vi "Begin.vi"() -> (0 "No error":errorcluster)   [LabVIEW 2012]
doc: "Called before other user functions, this VI is expected to open initial I/O refnums, load in file data, and do all program initialization. Notice that the <B>error out</B> terminal is simply used for data flow. Wiring it to other structures or subVIs ensures that this VI runs first."
panel:
  out "error out":errorcluster
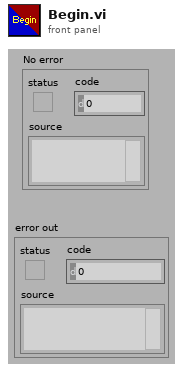
[diagram p1: front panel]
types:
  T1 = typedef "WPI_CameraDevRef.ctl" = cluster{"Camera Address":string, "CameraStatus":errorcluster, "Acquire Image Notifier":refnum<notifier>}
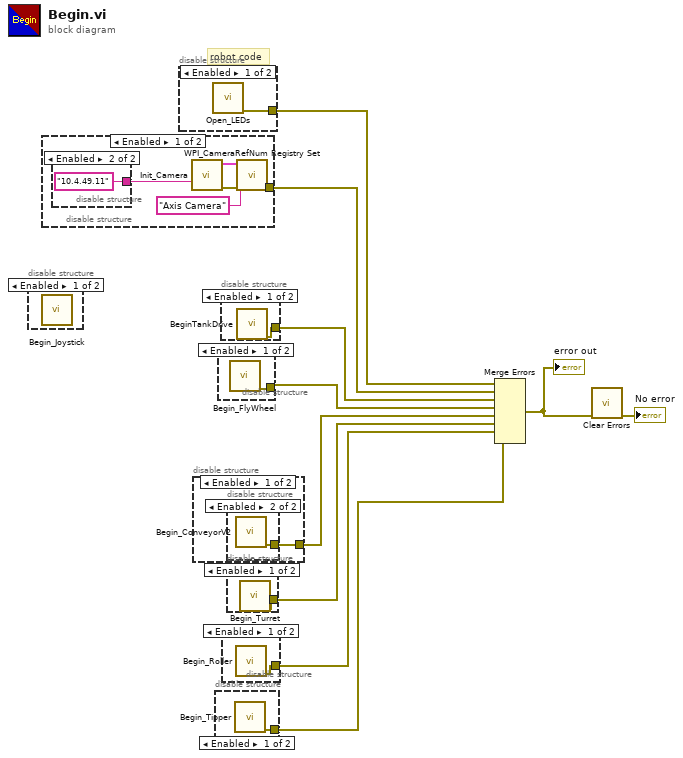
[diagram p0: block diagram]
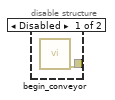
[diagram p7: hidden frame]
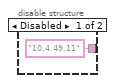
[diagram p10: hidden frame]
diagram:
  # "robot code"
  n1 = disable-structure shown="Enabled" {
    frame Enabled {
      n2 = call "Begin_Joystick.vi"() -> ()  [unwired: 12 in]
    }
    frame Disabled {
    }
  }
  n3 = disable-structure shown="Enabled" {
    disable-tunnel: [w11 _] -> w6
    frame Enabled {
      n4 = disable-structure shown="Enabled" {
        disable-tunnel: ["10.4.49.11" ("Camera IP") "10.4.49.11" ("Camera IP")] -> w15
        frame Disabled {
        }
        frame Enabled {
        }
      }
      n5 = call "Init_Camera.vi"("Camera IP"=w15) -> ("error out"=w12:errorcluster, "CameraDevRef Out"=w14:T1)  [unwired: 9 in]
      n6 = call <vilib>:"WPI_CameraRefNum Registry Set.vi"("error in (no error)"=w12, "refnum name"="Axis Camera", "CameraDevRef"=w14) -> ("error out"=w11:errorcluster)  [unwired: 7 in, 1 out]
    }
    frame Disabled {
    }
  }
  n7 = disable-structure shown="Enabled" {
    disable-tunnel: [w18 _] -> w5
    frame Enabled {
      n8 = call "Open_LEDs.vi"() -> ("error out"=w18:errorcluster)  [unwired: 10 in, 1 out]
    }
    frame Disabled {
    }
  }
  n9 = disable-structure shown="Enabled" {
    disable-tunnel: [w19 _] -> w10
    frame Enabled {
      n10 = disable-structure shown="Enabled" {
        disable-tunnel: [w20 w21] -> w19
        frame Disabled {
          n11 = call "begin_conveyor.vi"() -> ("error out"=w20:errorcluster)  [unwired: 11 in]
        }
        frame Enabled {
          n12 = call "Begin_ConveyorV2.vi"() -> ("error out"=w21:errorcluster)  [unwired: 11 in]
        }
      }
    }
    frame Disabled {
    }
  }
  n13 = disable-structure shown="Enabled" {
    disable-tunnel: [w22 _] -> w3
    frame Enabled {
      n14 = call "Begin_Tipper.vi"() -> ("error out"=w22:errorcluster)  [unwired: 11 in]
    }
    frame Disabled {
    }
  }
  n15 = disable-structure shown="Enabled" {
    disable-tunnel: [w23 _] -> w9
    frame Enabled {
      n16 = call "Begin_FlyWheel.vi"() -> ("error out"=w23:errorcluster)  [unwired: 11 in]
    }
    frame Disabled {
    }
  }
  n17 = disable-structure shown="Enabled" {
    disable-tunnel: [w24 _] -> w7
    frame Enabled {
      n18 = call "BeginTankDrive.vi"() -> ("error out"=w24:errorcluster)  [unwired: 11 in]
    }
    frame Disabled {
    }
  }
  n19 = disable-structure shown="Enabled" {
    disable-tunnel: [w25 _] -> w4
    frame Enabled {
      n20 = call "Begin_Roller.vi"() -> ("error out"=w25:errorcluster)  [unwired: 11 in]
    }
    frame Disabled {
    }
  }
  n21 = disable-structure shown="Enabled" {
    disable-tunnel: [w26 _] -> w8
    frame Enabled {
      n22 = call "Begin_Turret.vi"() -> ("error out"=w26:errorcluster)  [unwired: 11 in]
    }
    frame Disabled {
    }
  }
  n23 = Merge Errors(w5, w6, w7, w9, w10, w8, w4, w3) -> (w2:errorcluster)
  "error out" <- w2
  n24 = call <vilib>:"Clear Errors.vi"("error in (no error)"=w2) -> ("error out"=→"No error":errorcluster)  [unwired: 6 in]
